vi "Read Analogue.vi"(8 "error in (no error)":errorcluster, 11 "DMM in":refnum<class "NI DMM4072.lvclass">) -> (0 "error out":errorcluster, 2 "Measurement":dbl format="%.5f", 3 "DMM out":refnum<class "NI DMM4072.lvclass">)   [LabVIEW 2019, in "Concrete.lvlib" / "NI DMM4072.lvclass"]
uses:
  NI DMM4072.lvclass
  NI DMM4072.lvclass/NI DMM4072.ctl
  Harware Abstraction/MultiIO/MIO.lvclass
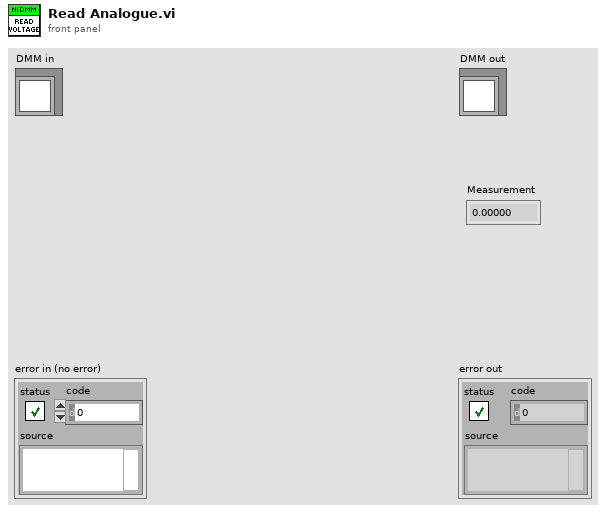
[diagram p1: front panel]
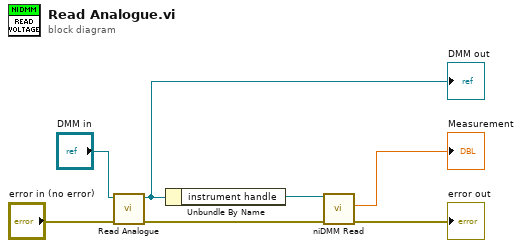
[diagram p0: block diagram]
diagram:
  n1 = call-parent "Read Analogue.vi"("error in (no error)"="error in (no error)", "DMM in"="DMM in") -> ("error out"=w5:errorcluster, "DMM out"=w3:refnum<class "NI DMM4072.lvclass">)  [unwired: 7 in, 1 out]
  "DMM out" <- w3
  n2 = Unbundle By Name(w3) -> ("instrument handle"=w2:refnum<k15>)
  n3 = call <instrlib>:"niDMM Read.vi"("error in (no error)"=w5, "instrument handle"=w2) -> ("error out"=→"error out":errorcluster, "Measurement"=→"Measurement":dbl)  [unwired: 7 in, 1 out]
